vi "Read Device Info.vi"() -> ()   [LabVIEW 2020]
uses:
  VisaResource/VisaResource.lvclass
  C:/dev/Vireo/PicoG/PicoG-Processor/PicoG-Core/DeployResource/DeployResource.lvclass
  DeployResource/DeployResource.lvclass
panel:
  out "Build":timestamp
  out "Version":string
  out "Alias":string
  out "ID":string
  out "Board":string
  out "Platform":string
  in  "VISA resource name":refnum<visa-resource-name>
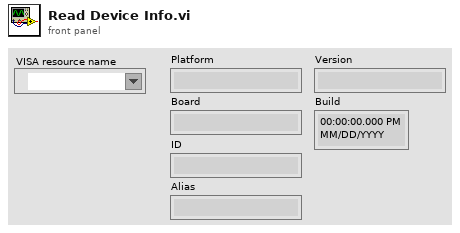
[diagram p1: front panel]
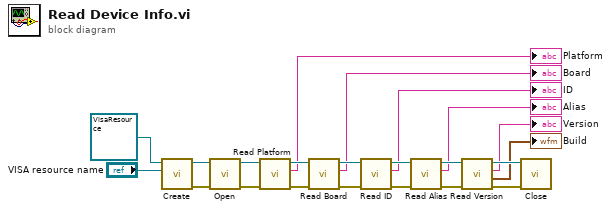
[diagram p0: block diagram]
diagram:
  n1 = call-dynamic "Create.vi"("Resource"="VISA resource name", "VisaResource in"=refnum<class "VisaResource.lvclass"> refnum) -> ("error out"=w19:errorcluster, "VisaResource out"=w20:refnum<class "VisaResource.lvclass">)  [unwired: 8 in]
  n2 = call-dynamic "Open.vi"("error in (no error)"=w19, "VisaResource in"=w20) -> ("error out"=w17:errorcluster, "VisaResource out"=w18:refnum<class "VisaResource.lvclass">)  [unwired: 8 in]
  n3 = call "Read Platform.vi"("error in (no error)"=w17, "DeployResource in"=w18) -> ("error out"=w15:errorcluster, "Platform"=→"Platform":string, "DeployResource out"=w16:refnum<class "VisaResource.lvclass">)  [unwired: 7 in]
  n4 = call "Read Board.vi"("error in (no error)"=w15, "DeployResource in"=w16) -> ("error out"=w13:errorcluster, "Board"=→"Board":string, "DeployResource out"=w14:refnum<class "VisaResource.lvclass">)  [unwired: 7 in]
  n5 = call "Read ID.vi"("error in (no error)"=w13, "DeployResource in"=w14) -> ("error out"=w11:errorcluster, "ID"=→"ID":string, "DeployResource out"=w12:refnum<class "VisaResource.lvclass">)  [unwired: 7 in]
  n6 = call "Read Alias.vi"("error in (no error)"=w11, "DeployResource in"=w12) -> ("error out"=w9:errorcluster, "Alias"=→"Alias":string, "DeployResource out"=w10:refnum<class "VisaResource.lvclass">)  [unwired: 7 in]
  n7 = call "Read Version.vi"("error in (no error)"=w9, "DeployResource in"=w10) -> ("error out"=w7:errorcluster, "Build"=→"Build":timestamp, "Version"=→"Version":string, "DeployResource out"=w8:refnum<class "VisaResource.lvclass">)  [unwired: 6 in]
  n8 = call-dynamic "Close.vi"("error in (no error)"=w7, "VisaResource in"=w8) -> ()  [unwired: 8 in, 2 out]
